vi "LibXML_GetNumberOfNodes.vi"(8 "error in (no error)":errorcluster, 11 "XPathObj":u32) -> (0 "error out":errorcluster, 2 "#ofNodes":i32, 3 "XPathObj out":u32)   [LabVIEW 2019, in "Tools.lvlib" / "LibXML.lvlib"]
doc: "Outputs the number of nodes in an XPath Object"
uses:
  LibXML.lvlib
  <vilib>/Utility/error.llb/Trim Whitespace.vi
  Tools.lvlib
  dll/lXMLwrap.dll
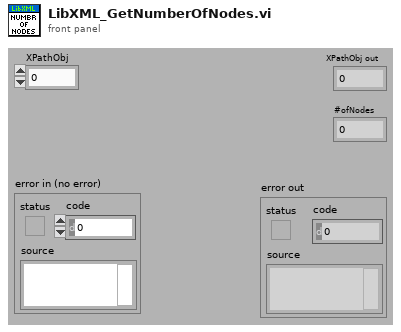
[diagram p1: front panel]
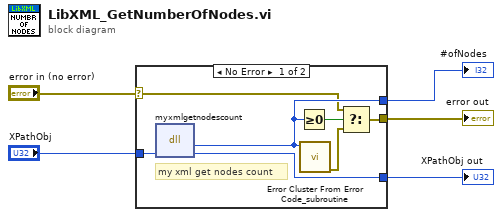
[diagram p0: block diagram]
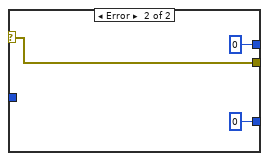
[diagram p2: hidden frame]
diagram:
  n1 = case shown="No Error" "error in (no error)" {
    selector: "error in (no error)" -> [w6 w15]
    tunnel: [w11 w15] -> w4
    tunnel: [w9 0] -> w3
    tunnel: "XPathObj" -> [w8 _]
    tunnel: [w7 u32 0 ("nodesetptr")] -> w1
    frame No Error {
      # "my xml get nodes count"
      n2 = dll-call lib="C:/Projects/_Prywatne/MyCIT/Framework/Tools/XML/LibXML/dll/lXMLwrap.dll" fn="myxmlgetnodescount"("nodesetptr"=w8) -> ("return type"=w9:i32, "nodesetptr"=w7:u32)  [unwired: 3 in, 2 out]
      n3 = Greater Or Equal To 0?(x=w9) -> (x >= 0?=w12:bool)
      n4 = call "Error Cluster From Error Code_subroutine.vi"("error code (0)"=w9) -> ("error out"=w10:errorcluster)  [unwired: 8 in]
      n5 = Select(t=w6, s=w12, f=w10) -> (s? t:f=w11:errorcluster)
    }
    frame Error {
    }
  }
  "error out" <- w4
  "#ofNodes" <- w3
  "XPathObj out" <- w1
